vi "Math-Increment Log Scale.vi"(0 "Old Value":dbl, 5 "Min":dbl, 7 "Max":dbl, 9 "Step":dbl, 11 "Increment":dbl) -> (4 "New Value":dbl)   [LabVIEW 2020]
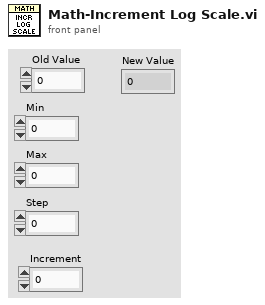
[diagram p1: front panel]
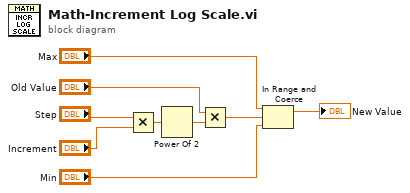
[diagram p0: block diagram]
diagram:
  n1 = Multiply(x="Step", y="Increment") -> (x*y=w9:dbl)
  n2 = Power Of 2(x=w9) -> (2^x=w8:dbl)
  n3 = Multiply(x="Old Value", y=w8) -> (x*y=w2:dbl)
  n4 = In Range and Coerce(upper limit="Max", x=w2, lower limit="Min") -> (coerced(x)=→"New Value":dbl)  [unwired: 1 out]
